vi "LuaVIEW Cast Gen Ref to VI Ref.vi"(7 "refnum in":refnum<vi>) -> (8 "refnum out":refnum<vi>)   [LabVIEW 2013]
doc: "This VI casts between incompatible refnum types. Refnums passed to Lua only carry their value and not their type. It is therefore required to cast them to a generic type on passing them to Lua and back from the generic type to their actual type on retrieval from Lua."
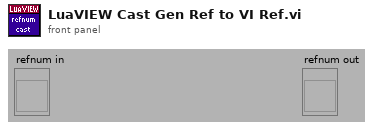
[diagram p1: front panel]
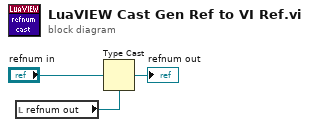
[diagram p0: block diagram]
diagram:
  n1 = local read "refnum out"() -> (w3:refnum<vi>)
  n2 = Type Cast(type=w3, x="refnum in") -> (*(type *) &x=→"refnum out":refnum<vi>)
